vi "Read dotNET Custom Action Definitions.vi"(8 "error in (no error)":errorcluster, 10 "Custom Action Definitions":refnum<k24>[](array[refnum]), 11 "Bundle Builder in":refnum<class "Bundle Builder.lvclass">) -> (0 "error out":errorcluster, 3 "Bundle Builder out":refnum<class "Bundle Builder.lvclass">)   [LabVIEW 2020, in "Bundle Builder.lvclass"]
uses:
  Bundle Builder.lvclass
  Bundle Builder.lvclass/Bundle Builder.ctl
  C:/Users/chihong/Documents/Repos/StsCustomBundleBuilder/Code/StsCustomBundleBuilder/StsCustomBundleBuilderLib/StsCustomBundleBuilderLib.dll
  StsCustomBundleBuilderLib/StsCustomBundleBuilderLib.dll
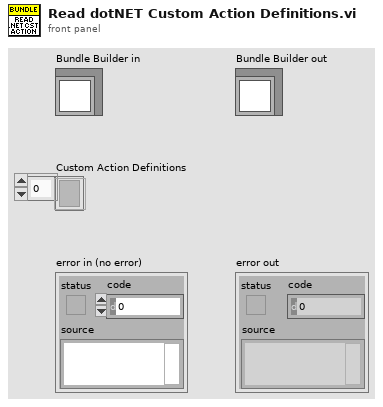
[diagram p1: front panel]
types:
  T1 = cluster{"Display Name":string, "Commands":cluster{"Path":string, "Parameters":string, "Successful Exit Codes":string}[]}
  T2 = cluster{"Path":string, "Parameters":string, "Successful Exit Codes":string}
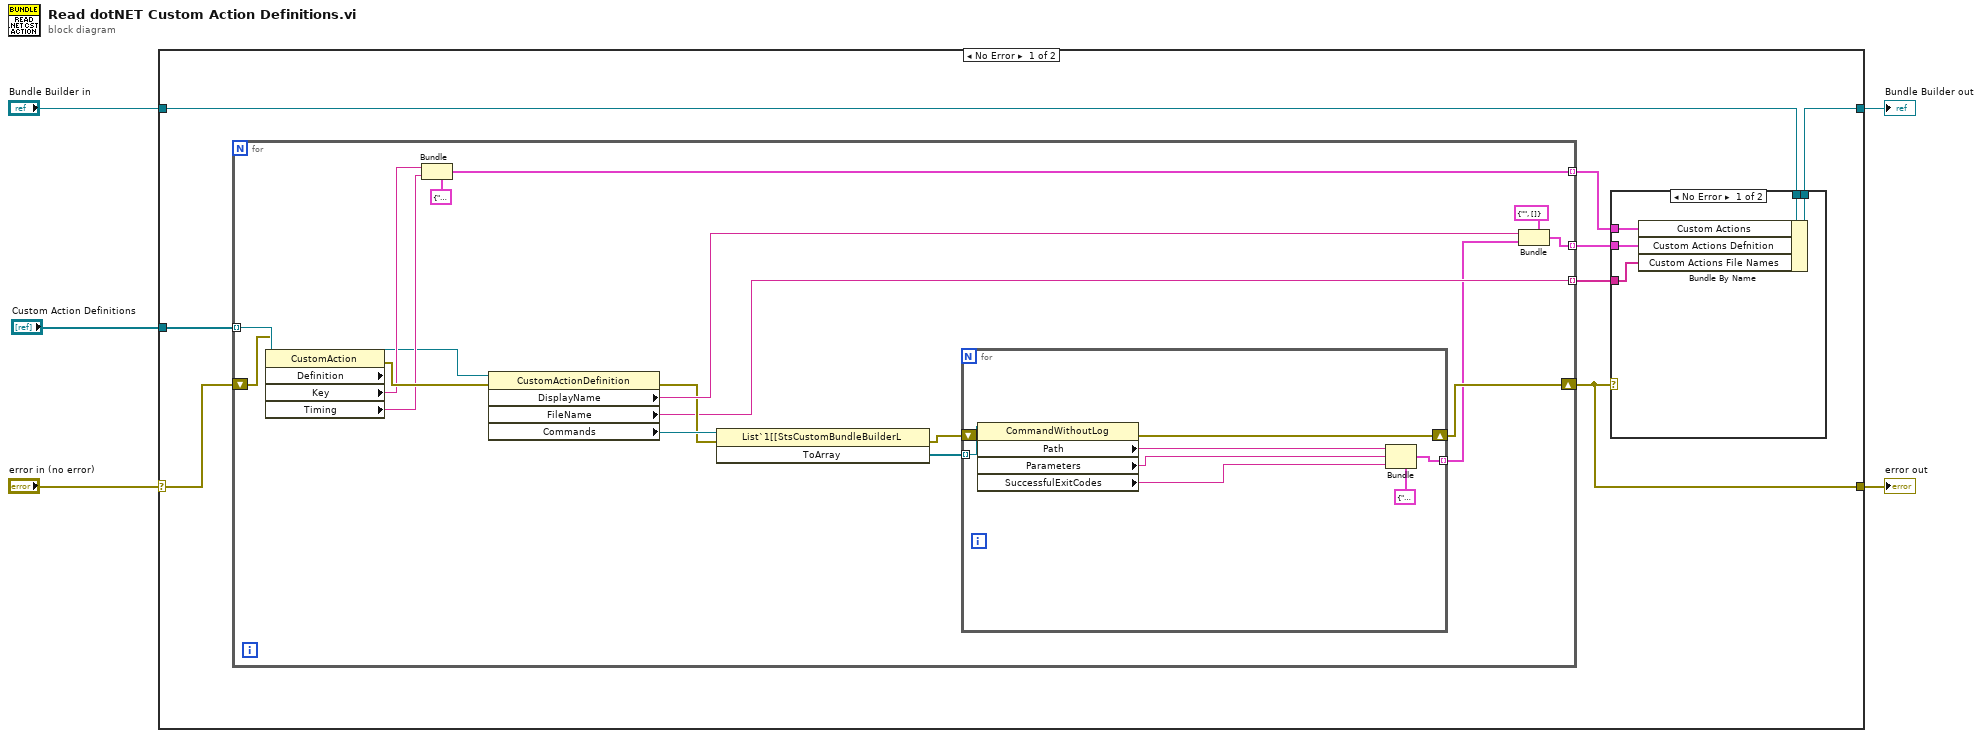
[diagram p0: block diagram]
diagram:
  n1 = case shown="No Error" "error in (no error)" {
    selector: "error in (no error)" -> [w11 w47]
    tunnel: [w7 w47] -> w4
    tunnel: [w10 w46] -> w2
    tunnel: "Bundle Builder in" -> [w13 w46]
    tunnel: "Custom Action Definitions" -> [w12 _]
    frame No Error {
      n2 = for {
        tunnel: w12 -> [w37] mode=indexing
        shift-right: [w26] -> w7
        shift-left: w11 -> [w36]
        tunnel: [w25] -> w9 mode=indexing
        tunnel: [w24] -> w8 mode=indexing
        tunnel: [w23] -> w6 mode=indexing
        n3 = property class="CustomAction"(reference=w37, error in=w36) -> (error out=w35:errorcluster, "Definition"=w32:refnum<k24>, "Key"=w34:string, "Timing"=w33:string)  [unwired: 1 out]
        n4 = Bundle(cluster=cluster{"Key":string, "Timing":string} {"Key"="", "Timing"=""} ("Product Installer"), "Key"=w34, "Timing"=w33) -> (w24:cluster{"Key":string, "Timing":string})
        n5 = property class="CustomActionDefinition"(reference=w32, error in=w35) -> (error out=w29:errorcluster, "DisplayName"=w31:string, "FileName"=w23:string, "Commands"=w30:refnum<k24>)  [unwired: 1 out]
        n6 = invoke class="List`1[[StsCustomBundleBuilderL" method="ToArray"(reference=w30, error in=w29) -> (error out=w27:errorcluster, "ToArray"=w28:refnum<k24>[])  [unwired: 1 in, 1 out]
        n7 = for {
          tunnel: w28 -> [w45] mode=indexing
          tunnel: [w39] -> w21 mode=indexing
          shift-right: [w42] -> w26
          shift-left: w27 -> [w41]
          n8 = property class="CommandWithoutLog"(reference=w45, error in=w41) -> (error out=w42:errorcluster, "Path"=w44:string, "Parameters"=w43:string, "SuccessfulExitCodes"=w40:string)  [unwired: 1 out]
          n9 = Bundle(cluster=T2 {"Path"="", "Parameters"="", "Successful Exit Codes"=""} ("Product Installer"), "Path"=w44, "Parameters"=w43, "Successful Exit Codes"=w40) -> (w39:T2)
        }
        n10 = Bundle(cluster=T1 {"Display Name"="", "Commands"=[]} ("Custom Actions"), "Display Name"=w31, "Commands"=w21) -> (w25:T1)
      }
      n11 = case shown="No Error" w7 {
        tunnel: w13 -> [w18 w19]
        tunnel: [w17 w19] -> w10
        tunnel: w9 -> [w14 _]
        tunnel: w8 -> [w16 _]
        tunnel: w6 -> [w15 _]
        frame No Error {
          n12 = Bundle By Name(cluster=w18, "Custom Actions"=w16, "Custom Actions Defnition"=w14, "Custom Actions File Names"=w15) -> (w17:refnum<class "Bundle Builder.lvclass">)
        }
        frame Error {
        }
      }
    }
    frame Error {
    }
  }
  "error out" <- w4
  "Bundle Builder out" <- w2
